vi "Weather Parse Test.vi"() -> ()   [LabVIEW 2020, in "CDM-Config.lvlib"] (continued)
                \"073355\"\n                    ],\n                    \"UGC\": [\n                        \"ANZ355\"\n                    ]\n                },\n                \"affectedZones\": [\n                    \"https://api.weather.gov/zones/forecast/ANZ355\"\n                ],\n                \"references\": [\n                    {\n                        \"@id\": \"https://api.weather.gov/alerts/urn:oid:2.49.0.1.840.0.65e698b6ba470dcf13b408ab2bfb144a0f90de6e.002.1\",\n                        \"identifier\": \"urn:oid:2.49.0.1.840.0.65e698b6ba470dcf13b408ab2bfb144a0f90de6e.002.1\",\n                        \"sender\": \"w-nws.webmaster@noaa.gov\",\n                        \"sent\": \"2025-12-03T03:02:00-05:00\"\n                    }\n                ],\n                \"sent\": \"2025-12-03T06:40:00-05:00\",\n                \"effective\": \"2025-12-03T06:40:00-05:00\",\n                \"onset\": \"2025-12-03T06:40:00-05:00\",\n                \"expires\": \"2025-12-03T12:00:00-05:00\",\n                \"ends\": \"2025-12-03T12:00:00-05:00\",\n                \"status\": \"Actual\",\n                \"messageType\": \"Update\",\n                \"category\": \"Met\",\n                \"severity\": \"Minor\",\n                \"certainty\": \"Likely\",\n                \"urgency\": \"Expected\",\n                \"event\": \"Small Craft Advisory\",\n                \"sender\": \"w-nws.webmaster@noaa.gov\",\n                \"senderName\": \"NWS Upton NY\",\n                \"headline\": \"Small Craft Advisory issued December 3 at 6:40AM EST until December 3 at 12:00PM EST by NWS Upton NY\",\n                \"description\": \"* WHAT...Northwest winds 10 to 20 kt with gusts up to 25 kt and\\nseas 3 to 5 feet.\\n\\n* WHERE...Sandy Hook NJ to Fire Island Inlet NY out 20 nm.\\n\\n* WHEN...Until noon EST today.\\n\\n* IMPACTS...Conditions will be hazardous to small craft.\",\n                \"instruction\": \"Inexperienced mariners, especially those operating smaller\\nvessels, should avoid navigating in hazardous conditions.\",\n                \"response\": \"Avoid\",\n                \"parameters\": {\n                    \"AWIPSidentifier\": [\n                        \"MWWOKX\"\n                    ],\n                    \"WMOidentifier\": [\n                        \"WHUS71 KOKX 031140\"\n                    ],\n                    \"NWSheadline\": [\n                        \"SMALL CRAFT ADVISORY REMAINS IN EFFECT UNTIL NOON EST TODAY\"\n                    ],\n                    \"BLOCKCHANNEL\": [\n                        \"EAS\",\n                        \"NWEM\",\n                        \"CMAS\"\n                    ],\n                    \"VTEC\": [\n                        \"/O.CON.KOKX.SC.Y.0111.000000T0000Z-251203T1700Z/\"\n                    ],\n                    \"eventEndingTime\": [\n                        \"2025-12-03T12:00:00-05:00\"\n                    ],\n                    \"expiredReferences\": [\n                        \"w-nws.webmaster@noaa.gov,urn:oid:2.49.0.1.840.0.ccba0ca9284c1e638a678cfbb9d4c4131fa82910.003.1,2025-12-02T13:01:00-05:00 w-nws.webmaster@noaa.gov,urn:oid:2.49.0.1.840.0.f66193c09c556463d3d8c63bce1b034f3b0ce6c5.001.1,2025-12-02T01:36:00-05:00 w-nws.webmaster@noaa.gov,urn:oid:2.49.0.1.840.0.57e44e37368416f721b2e96097448da44f0e554e.001.2,2025-12-01T13:22:00-05:00\"\n                    ]\n                },\n                \"scope\": \"Public\",\n                \"code\": \"IPAWSv1.0\",\n                \"language\": \"en-US\",\n                \"web\": \"http://www.weather.gov\",\n                \"eventCode\": {\n                    \"SAME\": [\n                        \"NWS\"\n                    ],\n                    \"NationalWeatherService\": [\n                        \"SCY\"\n                    ]\n                }\n            }\n        },\n        {\n            \"id\": \"https://api.weather.gov/alerts/urn:oid:2.49.0.1.840.0.eda6a12a51dab3b83bf60aa6decb3c42e9ebbac9.001.2\",\n            \"type\": \"Feature\",\n            \"geometry\": null,\n            \"properties\": {\n                \"@id\": \"https://api.weather.gov/alerts/urn:oid:2.49.0.1.840.0.eda6a12a51dab3b83bf60aa6decb3c42e9ebbac9.001.2\",\n                \"@type\": \"wx:Alert\",\n                \"id\": \"urn:oid:2.49.0.1.840.0.eda6a12a51dab3b83bf60aa6decb3c42e9ebbac9.001.2\",\n                \"areaDesc\": \"Moriches Inlet NY to Montauk Point NY out 20 nm; Fire Island Inlet NY to Moriches Inlet NY out 20 nm\",\n                \"geocode\": {\n                    \"SAME\": [\n                        \"073350\",\n                        \"073353\"\n                    ],\n                    \"UGC\": [\n                        \"ANZ350\",\n                        \"ANZ353\"\n                    ]\n                },\n                \"affectedZones\": [\n                    \"https://api.weather.gov/zones/forecast/ANZ350\",\n                    \"https://api.weather.gov/zones/forecast/ANZ353\"\n                ],\n                \"references\": [\n                    {\n                        \"@id\": \"https://api.weather.gov/alerts/urn:oid:2.49.0.1.840.0.65e698b6ba470dcf13b408ab2bfb144a0f90de6e.001.2\",\n                        \"identifier\": \"urn:oid:2.49.0.1.840.0.65e698b6ba470dcf13b408ab2bfb144a0f90de6e.001.2\",\n                        \"sender\": \"w-nws.webmaster@noaa.gov\",\n                        \"sent\": \"2025-12-03T03:02:00-05:00\"\n                    }\n                ],\n                \"sent\": \"2025-12-03T06:40:00-05:00\",\n                \"effective\": \"2025-12-03T06:40:00-05:00\",\n                \"onset\": \"2025-12-04T15:00:00-05:00\",\n                \"expires\": \"2025-12-03T19:45:00-05:00\",\n                \"ends\": \"2025-12-05T06:00:00-05:00\",\n                \"status\": \"Actual\",\n                \"messageType\": \"Update\",\n                \"category\": \"Met\",\n                \"severity\": \"Moderate\",\n                \"certainty\": \"Possible\",\n                \"urgency\": \"Future\",\n                \"event\": \"Gale Watch\",\n                \"sender\": \"w-nws.webmaster@noaa.gov\",\n                \"senderName\": \"NWS Upton NY\",\n                \"headline\": \"Gale Watch issued December 3 at 6:40AM EST until December 5 at 6:00AM EST by NWS Upton NY\",\n                \"description\": \"* WHAT...For the Small Craft Advisory, west winds 15 to 20 kt with\\ngusts up to 25 kt and seas 4 to 7 feet. For the Gale Watch,\\nnorthwest winds 20 to 30 kt with gusts up to 40 kt and seas 5 to\\n8 feet possible.\\n\\n* WHERE...Fire Island Inlet NY to Montauk Point NY out 20 nm.\\n\\n* WHEN...For the Small Craft Advisory, until 3 PM EST Thursday.\\nFor the Gale Watch, from Thursday afternoon through late\\nThursday night.\\n\\n* IMPACTS...Strong winds can cause hazardous seas which could\\ncapsize or damage vessels and reduce visibility.\",\n                \"instruction\": \"Mariners should consider altering plans to avoid possible\\nhazardous conditions.  Remain in port, seek safe harbor, alter\\ncourse, and/or secure the vessel for severe wind and seas.\",\n                \"response\": \"Prepare\",\n                \"parameters\": {\n                    \"AWIPSidentifier\": [\n                        \"MWWOKX\"\n                    ],\n                    \"WMOidentifier\": [\n                        \"WHUS71 KOKX 031140\"\n                    ],\n                    \"NWSheadline\": [\n                        \"SMALL CRAFT ADVISORY REMAINS IN EFFECT UNTIL 3 PM EST THURSDAY... ...GALE WATCH REMAINS IN EFFECT FROM THURSDAY AFTERNOON THROUGH LATE THURSDAY NIGHT\"\n                    ],\n                    \"BLOCKCHANNEL\": [\n                        \"EAS\",\n                        \"NWEM\",\n                        \"CMAS\"\n                    ],\n                    \"VTEC\": [\n                        \"/O.CON.KOKX.GL.A.0021.251204T2000Z-251205T1100Z/\"\n                    ],\n                    \"eventEndingTime\": [\n                        \"2025-12-05T06:00:00-05:00\"\n                    ]\n                },\n                \"scope\": \"Public\",\n                \"code\": \"IPAWSv1.0\",\n                \"language\": \"en-US\",\n                \"web\": \"http://www.weather.gov\",\n                \"eventCode\": {\n                    \"SAME\": [\n                        \"NWS\"\n                    ],\n                    \"NationalWeatherService\": [\n                        \"GLA\"\n                    ]\n                }\n            }\n        },\n        {\n            \"id\": \"https://api.weather.gov/alerts/urn:oid:2.49.0.1.840.0.0d83c610c5424770356d8de2248dc8d571fcc2f4.001.1\",\n            \"type\": \"Feature\",\n            \"geometry\": null,\n            \"properties\": {\n                \"@id\": \"https://api.weather.gov/alerts/urn:oid:2.49.0.1.840.0.0d83c610c5424770356d8de2248dc8d571fcc2f4.001.1\",\n                \"@type\": \"wx:Alert\",\n                \"id\": \"urn:oid:2.49.0.1.840.0.0d83c610c5424770356d8de2248dc8d571fcc2f4.001.1\",\n                \"areaDesc\": \"Foothills of the Northern Blue Mountains of Oregon; Yakima Valley; Foothills of the Blue Mountains of Washington\",\n                \"geocode\": {\n                    \"SAME\": [\n                        \"041059\",\n                        \"053077\",\n                        \"053013\",\n                        \"053071\"\n                    ],\n                    \"UGC\": [\n                        \"ORZ507\",\n                        \"WAZ027\",\n                        \"WAZ029\"\n                    ]\n                },\n                \"affectedZones\": [\n                    \"https://api.weather.gov/zones/forecast/ORZ507\",\n                    \"https://api.weather.gov/zones/forecast/WAZ027\",\n                    \"https://api.weather.gov/zones/forecast/WAZ029\"\n                ],\n                \"references\": [],\n                \"sent\": \"2025-12-03T02:34:00-08:00\",\n                \"effective\": \"2025-12-03T02:34:00-08:00\",\n                \"onset\": \"2025-12-03T02:34:00-08:00\",\n                \"expires\": \"2025-12-03T10:00:00-08:00\",\n                \"ends\": \"2025-12-03T10:00:00-08:00\",\n                \"status\": \"Actual\",\n                \"messageType\": \"Alert\",\n                \"category\": \"Met\",\n                \"severity\": \"Moderate\",\n                \"certainty\": \"Likely\",\n                \"urgency\": \"Expected\",\n                \"event\": \"Freezing Fog Advisory\",\n                \"sender\": \"w-nws.webmaster@noaa.gov\",\n                \"senderName\": \"NWS Pendleton OR\",\n                \"headline\": \"Freezing Fog Advisory issued December 3 at 2:34AM PST until December 3 at 10:00AM PST by NWS Pendleton OR\",\n                \"description\": \"* WHAT...Visibility generally between one-half mile and one mile in\\nfog and freezing fog.\\n\\n* WHERE...In Oregon, Foothills of the Northern Blue Mountains of\\nOregon. In Washington, Yakima Valley and Foothills of the Blue\\nMountains of Washington.\\n\\n* WHEN...Until 10 AM PST this morning.\\n\\n* IMPACTS...Low visibility could make driving conditions hazardous.\\n\\n* ADDITIONAL DETAILS...Webcams show reduced visibilities on portions\\nof I-84, SR-204 and SR-11 near Pendleton, Athena and Walla Walla\\nand SR-24 and I-82 between Sunnyside and Yakima.\",\n                \"instruction\": \"If driving, slow down, use low beam headlights, and leave plenty of\\ndistance ahead of you.\",\n                \"response\": \"Avoid\",\n                \"parameters\": {\n                    \"AWIPSidentifier\": [\n                        \"NPWPDT\"\n                    ],\n                    \"WMOidentifier\": [\n                        \"WWUS76 KPDT 031034\"\n                    ],\n                    \"NWSheadline\": [\n                        \"FREEZING FOG ADVISORY IN EFFECT UNTIL 10 AM PST THIS MORNING\"\n                    ],\n                    \"BLOCKCHANNEL\": [\n                        \"EAS\",\n                        \"NWEM\",\n                        \"CMAS\"\n                    ],\n                    \"VTEC\": [\n                        \"/O.NEW.KPDT.ZF.Y.0011.251203T1034Z-251203T1800Z/\"\n                    ],\n                    \"eventEndingTime\": [\n                        \"2025-12-03T10:00:00-08:00\"\n                    ]\n                },\n                \"scope\": \"Public\",\n                \"code\": \"IPAWSv1.0\",\n                \"language\": \"en-US\",\n                \"web\": \"http://www.weather.gov\",\n                \"eventCode\": {\n                    \"SAME\": [\n                        \"NWS\"\n                    ],\n                    \"NationalWeatherService\": [\n                        \"ZFY\"\n                    ]\n                }\n            }\n        },\n        {\n            \"id\": \"https://api.weather.gov/alerts/urn:oid:2.49.0.1.840.0.15f495c3cdd4a42513043897320797e7c1790118.004.1\",\n            \"type\": \"Feature\",\n            \"geometry\": null,\n            \"properties\": {\n                \"@id\": \"https://api.weather.gov/alerts/urn:oid:2.49.0.1.840.0.15f495c3cdd4a42513043897320797e7c1790118.004.1\",\n                \"@type\": \"wx:Alert\",\n                \"id\": \"urn:oid:2.49.0.1.840.0.15f495c3cdd4a42513043897320797e7c1790118.004.1\",\n                \"areaDesc\": \"Waters from Point Pinos to Point Piedras Blancas 10-60 NM\",\n                \"geocode\": {\n                    \"SAME\": [\n                        \"057576\"\n                    ],\n                    \"UGC\": [\n                        \"PZZ576\"\n                    ]\n                },\n                \"affectedZones\": [\n                    \"https://api.weather.gov/zones/forecast/PZZ576\"\n                ],\n                \"references\": [\n                    {\n                        \"@id\": \"https://api.weather.gov/alerts/urn:oid:2.49.0.1.840.0.2e2b4d19d93828c0d7fe64253ee2ca5ea893eca3.004.1\",\n                        \"identifier\": \"urn:oid:2.49.0.1.840.0.2e2b4d19d93828c0d7fe64253ee2ca5ea893eca3.004.1\",\n                        \"sender\": \"w-nws.webmaster@noaa.gov\",\n                        \"sent\": \"2025-12-02T20:09:00-08:00\"\n                    }\n                ],\n                \"sent\": \"2025-12-03T02:34:00-08:00\",\n                \"effective\": \"2025-12-03T02:34:00-08:00\",\n                \"onset\": \"2025-12-03T02:34:00-08:00\",\n                \"expires\": \"2025-12-03T09:00:00-08:00\",\n                \"ends\": \"2025-12-03T09:00:00-08:00\",\n                \"status\": \"Actual\",\n                \"messageType\": \"Update\",\n                \"category\": \"Met\",\n                \"severity\": \"Minor\",\n                \"certainty\": \"Likely\",\n                \"urgency\": \"Expected\",\n                \"event\": \"Small Craft Advisory\",\n                \"sender\": \"w-nws.webmaster@noaa.gov\",\n                \"senderName\": \"NWS San Francisco CA\",\n                \"headline\": \"Small Craft Advisory issued December 3 at 2:34AM PST until December 3 at 9:00AM PST by NWS San Francisco CA\",\n                \"description\": \"* WHAT...North winds 15 to 20 kt with gusts up to 30 kt and seas\\n8 to 10 ft.\\n\\n* WHERE...Waters from Point Pinos to Point Piedras Blancas 10-\\n60 NM.\\n\\n* WHEN...Until 9 AM PST this morning.\\n\\n* IMPACTS...Conditions will be hazardous to small craft.\",\n                \"instruction\": \"Inexperienced mariners, especially those operating smaller\\nvessels, should avoid navigating in hazardous conditions.\",\n                \"response\": \"Avoid\",\n                \"parameters\": {\n                    \"AWIPSidentifier\": [\n                        \"MWWMTR\"\n                    ],\n                    \"WMOidentifier\": [\n                        \"WHUS76 KMTR 031034\"\n                    ],\n                    \"NWSheadline\": [\n                        \"SMALL CRAFT ADVISORY NOW IN EFFECT UNTIL 9 AM PST THIS MORNING\"\n                    ],\n                    \"BLOCKCHANNEL\": [\n                        \"EAS\",\n                        \"NWEM\",\n                        \"CMAS\"\n                    ],\n                    \"VTEC\": [\n                        \"/O.EXT.KMTR.SC.Y.0211.000000T0000Z-251203T1700Z/\"\n                    ],\n                    \"eventEndingTime\": [\n                        \"2025-12-03T09:00:00-08:00\"\n                    ],\n                    \"expiredReferences\": [\n                        \"w-nws.webmaster@noaa.gov,urn:oid:2.49.0.1.840.0.9218f4c28c3a850a1d7ea8eb0351e78dfe99a87f.003.1,2025-12-02T14:32:00-08:00 w-nws.webmaster@noaa.gov,urn:oid:2.49.0.1.840.0.0694ec14bef3aec9c3b54940004682f896b5d224.006.1,2025-12-02T08:49:00-08:00 w-nws.webmaster@noaa.gov,urn:oid:2.49.0.1.840.0.917c99b05a9fd34906c56c3461dc077eb8fbc6c3.005.1,2025-12-02T02:30:00-08:00 w-nws.webmaster@noaa.gov,urn:oid:2.49.0.1.840.0.71e8f8c0a9680225e124435739f52670c4652e60.005.1,2025-12-01T20:36:00-08:00 w-nws.webmaster@noaa.gov,urn:oid:2.49.0.1.840.0.dc88dd948d918d864c0dc5e6ad60facca6edd43a.003.1,2025-12-01T14:02:00-08:00\"\n                    ]\n                },\n                \"scope\": \"Public\",\n                \"code\": \"IPAWSv1.0\",\n                \"language\": \"en-US\",\n                \"web\": \"http://www.weather.gov\",\n                \"eventCode\": {\n                    \"SAME\": [\n                        \"NWS\"\n                    ],\n                    \"NationalWeatherService\": [\n                        \"SCY\"\n                    ]\n                }\n            }\n        },\n        {\n            \"id\": \"https://api.weather.gov/alerts/urn:oid:2.49.0.1.840.0.15f495c3cdd4a42513043897320797e7c1790118.003.1\",\n            \"type\": \"Feature\",\n            \"geometry\": null,\n            \"properties\": {\n                \"@id\": \"https://api.weather.gov/alerts/urn:oid:2.49.0.1.840.0.15f495c3cdd4a42513043897320797e7c1790118.003.1\",\n                \"@type\": \"wx:Alert\",\n                \"id\": \"urn:oid:2.49.0.1.840.0.15f495c3cdd4a42513043897320797e7c1790118.003.1\",\n                \"areaDesc\": \"Waters from Point Reyes to Pigeon Point 10-60 NM\",\n                \"geocode\": {\n                    \"SAME\": [\n                        \"057571\"\n                    ],\n                    \"UGC\": [\n                        \"PZZ571\"\n                    ]\n                },\n                \"affectedZones\": [\n                    \"https://api.weather.gov/zones/forecast/PZZ571\"\n                ],\n                \"references\": [\n                    {\n                        \"@id\": \"https://api.weather.gov/alerts/urn:oid:2.49.0.1.840.0.2e2b4d19d93828c0d7fe64253ee2ca5ea893eca3.002.1\",\n                        \"identifier\": \"urn:oid:2.49.0.1.840.0.2e2b4d19d93828c0d7fe64253ee2ca5ea893eca3.002.1\",\n                        \"sender\": \"w-nws.webmaster@noaa.gov\",\n                        \"sent\": \"2025-12-02T20:09:00-08:00\"\n                    }\n                ],\n                \"sent\": \"2025-12-03T02:34:00-08:00\",\n                \"effective\": \"2025-12-03T02:34:00-08:00\",\n                \"onset\": \"2025-12-03T02:34:00-08:00\",\n                \"expires\": \"2025-12-03T10:45:00-08:00\",\n                \"ends\": \"2025-12-03T09:00:00-08:00\",\n                \"status\": \"Actual\",\n                \"messageType\": \"Update\",\n                \"category\": \"Met\",\n                \"severity\": \"Minor\",\n                \"certainty\": \"Likely\",\n                \"urgency\": \"Expected\",\n                \"event\": \"Small Craft Advisory\",\n                \"sender\": \"w-nws.webmaster@noaa.gov\",\n                \"senderName\": \"NWS San Francisco CA\",\n                \"headline\": \"Small Craft Advisory issued December 3 at 2:34AM PST until December 3 at 9:00AM PST by NWS San Francisco CA\",\n                \"description\": \"* WHAT...For the first Small Craft Advisory, north winds 10 to\\n20 kt with gusts up to 30 kt and seas 8 to 11 ft. For the\\nsecond Small Craft Advisory, northwest winds 10 to 20 kt with\\ngusts up to 30 kt expected.\\n\\n* WHERE...Waters from Point Reyes to Pigeon Point 10-60 NM.\\n\\n* WHEN...For the first Small Craft Advisory, until 9 AM PST this\\nmorning. For the second Small Craft Advisory, from 9 PM\\nThursday to 9 AM PST Friday.\\n\\n* IMPACTS...Conditions will be hazardous to small craft.\",\n                \"instruction\": \"Inexperienced mariners, especially those operating smaller\\nvessels, should avoid navigating in hazardous conditions.\",\n                \"response\": \"Avoid\",\n                \"parameters\": {\n                    \"AWIPSidentifier\": [\n                        \"MWWMTR\"\n                    ],\n                    \"WMOidentifier\": [\n                        \"WHUS76 KMTR 031034\"\n                    ],\n                    \"NWSheadline\": [\n                        \"SMALL CRAFT ADVISORY REMAINS IN EFFECT UNTIL 9 AM PST THIS MORNING... ...SMALL CRAFT ADVISORY IN EFFECT FROM 9 PM THURSDAY TO 9 AM PST FRIDAY\"\n                    ],\n                    \"BLOCKCHANNEL\": [\n                        \"EAS\",\n                        \"NWEM\",\n                        \"CMAS\"\n                    ],\n                    \"VTEC\": [\n                        \"/O.CON.KMTR.SC.Y.0210.000000T0000Z-251203T1700Z/\"\n                    ],\n                    \"eventEndingTime\": [\n                        \"2025-12-03T09:00:00-08:00\"\n                    ],\n                    \"expiredReferences\": [\n                        \"w-nws.webmaster@noaa.gov,urn:oid:2.49.0.1.840.0.9218f4c28c3a850a1d7ea8eb0351e78dfe99a87f.004.1,2025-12-02T14:32:00-08:00 w-nws.webmaster@noaa.gov,urn:oid:2.49.0.1.840.0.0694ec14bef3aec9c3b54940004682f896b5d224.003.1,2025-12-02T08:49:00-08:00 w-nws.webmaster@noaa.gov,urn:oid:2.49.0.1.840.0.917c99b05a9fd34906c56c3461dc077eb8fbc6c3.003.1,2025-12-02T02:30:00-08:00 w-nws.webmaster@noaa.gov,urn:oid:2.49.0.1.840.0.71e8f8c0a9680225e124435739f52670c4652e60.002.1,2025-12-01T20:36:00-08:00 w-nws.webmaster@noaa.gov,urn:oid:2.49.0.1.840.0.dc88dd948d918d864c0dc5e6ad60facca6edd43a.004.1,2025-12-01T14:02:00-08:00\"\n                    ]\n                },\n                \"scope\": \"Public\",\n                \"code\": \"IPAWSv1.0\",\n                \"language\": \"en-US\",\n                \"web\": \"http://www.weather.gov\",\n                \"eventCode\": {\n                    \"SAME\": [\n                        \"NWS\"\n                    ],\n                    \"NationalWeatherService\": [\n                        \"SCY\"\n                    ]\n                }\n            }\n        },\n        {\n            \"id\": \"https://api.weather.gov/alerts/urn:oid:2.49.0.1.840.0.15f495c3cdd4a42513043897320797e7c1790118.003.2\",\n            \"type\": \"Feature\",\n            \"geometry\": null,\n            \"properties\": {\n                \"@id\": \"https://api.weather.gov/alerts/urn:oid:2.49.0.1.840.0.15f495c3cdd4a42513043897320797e7c1790118.003.2\",\n                \"@type\": \"wx:Alert\",\n                \"id\": \"urn:oid:2.49.0.1.840.0.15f495c3cdd4a42513043897320797e7c1790118.003.2\",\n                \"areaDesc\": \"Waters from Point Reyes to Pigeon Point 10-60 NM\",\n                \"geocode\": {\n                    \"SAME\": [\n                        \"057571\"\n                    ],\n                    \"UGC\": [\n                        \"PZZ571\"\n                    ]\n                },\n                \"affectedZones\": [\n                    \"https://api.weather.gov/zones/forecast/PZZ571\"\n                ],\n                \"references\": [],\n                \"sent\": \"2025-12-03T02:34:00-08:00\",\n                \"effective\": \"2025-12-03T02:34:00-08:00\",\n                \"onset\": \"2025-12-04T21:00:00-08:00\",\n                \"expires\": \"2025-12-03T10:45:00-08:00\",\n                \"ends\": \"2025-12-05T09:00:00-08:00\",\n                \"status\": \"Actual\",\n                \"messageType\": \"Alert\",\n                \"category\": \"Met\",\n                \"severity\": \"Minor\",\n                \"certainty\": \"Likely\",\n                \"urgency\": \"Expected\",\n                \"event\": \"Small Craft Advisory\",\n                \"sender\": \"w-nws.webmaster@noaa.gov\",\n                \"senderName\": \"NWS San Francisco CA\",\n                \"headline\": \"Small Craft Advisory issued December 3 at 2:34AM PST until December 5 at 9:00AM PST by NWS San Francisco CA\",\n                \"description\": \"* WHAT...For the first Small Craft Advisory, north winds 10 to\\n20 kt with gusts up to 30 kt and seas 8 to 11 ft. For the\\nsecond Small Craft Advisory, northwest winds 10 to 20 kt with\\ngusts up to 30 kt expected.\\n\\n* WHERE...Waters from Point Reyes to Pigeon Point 10-60 NM.\\n\\n* WHEN...For the first Small Craft Advisory, until 9 AM PST this\\nmorning. For the second Small Craft Advisory, from 9 PM\\nThursday to 9 AM PST Friday.\\n\\n* IMPACTS...Conditions will be hazardous to small craft.\",\n                \"instruction\": \"Inexperienced mariners, especially those operating smaller\\nvessels, should avoid navigating in hazardous conditions.\",\n                \"response\": \"Avoid\",\n                \"parameters\": {\n                    \"AWIPSidentifier\": [\n                        \"MWWMTR\"\n                    ],\n                    \"WMOidentifier\": [\n                        \"WHUS76 KMTR 031034\"\n                    ],\n                    \"NWSheadline\": [\n                        \"SMALL CRAFT ADVISORY REMAINS IN EFFECT UNTIL 9 AM PST THIS MORNING... ...SMALL CRAFT ADVISORY IN EFFECT FROM 9 PM THURSDAY TO 9 AM PST FRIDAY\"\n                    ],\n                    \"BLOCKCHANNEL\": [\n                        \"EAS\",\n                        \"NWEM\",\n                        \"CMAS\"\n                    ],\n                    \"VTEC\": [\n                        \"/O.NEW.KMTR.SC.Y.0212.251205T0500Z-251205T1700Z/\"\n                    ],\n                    \"eventEndingTime\": [\n                        \"2025-12-05T09:00:00-08:00\"\n                    ]\n                },\n                \"scope\": \"Public\",\n                \"code\": \"IPAWSv1.0\",\n                \"language\": \"en-US\",\n                \"web\": \"http://www.weather.gov\",\n                \"eventCode\": {\n                    \"SAME\": [\n                        \"NWS\"\n                    ],\n                    \"NationalWeatherService\": [\n                        \"SCY\"\n                    ]\n                }\n            }\n        },\n        {\n            \"id\": \"https://api.weather.gov/alerts/urn:oid:2.49.0.1.840.0.15f495c3cdd4a42513043897320797e7c1790118.002.2\",\n            \"type\": \"Feature\",\n            \"geometry\": null,\n            \"properties\": {\n                \"@id\": \"https://api.weather.gov/alerts/urn:oid:2.49.0.1.840.0.15f495c3cdd4a42513043897320797e7c1790118.002.2\",\n                \"@type\": \"wx:Alert\",\n                \"id\": \"urn:oid:2.49.0.1.840.0.15f495c3cdd4a42513043897320797e7c1790118.002.2\",\n                \"areaDesc\": \"Waters from Point Arena to Point Reyes 10-60 NM\",\n                \"geocode\": {\n                    \"SAME\": [\n                        \"057570\"\n                    ],\n                    \"UGC\": [\n                        \"PZZ570\"\n                    ]\n                },\n                \"affectedZones\": [\n                    \"https://api.weather.gov/zones/forecast/PZZ570\"\n                ],\n                \"references\": [],\n                \"sent\": \"2025-12-03T02:34:00-08:00\",\n                \"effective\": \"2025-12-03T02:34:00-08:00\",\n                \"onset\": \"2025-12-04T21:00:00-08:00\",\n                \"expires\": \"2025-12-03T10:45:00-08:00\",\n                \"ends\": \"2025-12-05T09:00:00-08:00\",\n                \"status\": \"Actual\",\n                \"messageType\": \"Alert\",\n                \"category\": \"Met\",\n                \"severity\": \"Minor\",\n                \"certainty\": \"Likely\",\n                \"urgency\": \"Expected\",\n                \"event\": \"Small Craft Advisory\",\n                \"sender\": \"w-nws.webmaster@noaa.gov\",\n                \"senderName\": \"NWS San Francisco CA\",\n                \"headline\": \"Small Craft Advisory issued December 3 at 2:34AM PST until December 5 at 9:00AM PST by NWS San Francisco CA\",\n                \"description\": \"* WHAT...For the first Small Craft Advisory, north winds 15 to\\n25 kt with gusts up to 35 kt and seas 8 to 11 ft. For the\\nsecond Small Craft Advisory, north winds 15 to 25 kt with\\ngusts up to 30 kt expected.\\n\\n* WHERE...Waters from Point Arena to Point Reyes 10-60 NM.\\n\\n* WHEN...For the first Small Craft Advisory, until 3 PM PST this\\nafternoon. For the second Small Craft Advisory, from 9 PM\\nThursday to 9 AM PST Friday.\\n\\n* IMPACTS...Conditions will be hazardous to small craft.\",\n                \"instruction\": \"Inexperienced mariners, especially those operating smaller\\nvessels, should avoid navigating in hazardous conditions.\",\n                \"response\": \"Avoid\",\n                \"parameters\": {\n                    \"AWIPSidentifier\": [\n                        \"MWWMTR\"\n                    ],\n                    \"WMOidentifier\": [\n                        \"WHUS76 KMTR 031034\"\n                    ],\n                    \"NWSheadline\": [\n                        \"SMALL CRAFT ADVISORY REMAINS IN EFFECT UNTIL 3 PM PST THIS AFTERNOON... ...SMALL CRAFT ADVISORY IN EFFECT FROM 9 PM THURSDAY TO 9 AM PST FRIDAY\"\n                    ],\n                    \"BLOCKCHANNEL\": [\n                        \"EAS\",\n                        \"NWEM\",\n                        \"CMAS\"\n                    ],\n                    \"VTEC\": [\n                        \"/O.NEW.KMTR.SC.Y.0212.251205T0500Z-251205T1700Z/\"\n                    ],\n                    \"eventEndingTime\": [\n                        \"2025-12-05T09:00:00-08:00\"\n                    ]\n                },\n                \"scope\": \"Public\",\n                \"code\": \"IPAWSv1.0\",\n                \"language\": \"en-US\",\n                \"web\": \"http://www.weather.gov\",\n                \"eventCode\": {\n                    \"SAME\": [\n                        \"NWS\"\n                    ],\n                    \"NationalWeatherService\": [\n                        \"SCY\"\n                    ]\n                }\n            }\n        },\n        {\n            \"id\": \"https://api.weather.gov/alerts/urn:oid:2.49.0.1.840.0.15f495c3cdd4a42513043897320797e7c1790118.002.1\",\n            \"type\": \"Feature\",\n            \"geometry\": null,\n            \"properties\": {\n                \"@id\": \"https://api.weather.gov/alerts/urn:oid:2.49.0.1.840.0.15f495c3cdd4a42513043897320797e7c1790118.002.1\",\n                \"@type\": \"wx:Alert\",\n                \"id\": \"urn:oid:2.49.0.1.840.0.15f495c3cdd4a42513043897320797e7c1790118.002.1\",\n                \"areaDesc\": \"Waters from Point Arena to Point Reyes 10-60 NM\",\n                \"geocode\": {\n                    \"SAME\": [\n                        \"057570\"\n                    ],\n                    \"UGC\": [\n                        \"PZZ570\"\n                    ]\n                },\n                \"affectedZones\": [\n                    \"https://api.weather.gov/zones/forecast/PZZ570\"\n                ],\n                \"references\": [\n                    {\n                        \"@id\": \"https://api.weather.gov/alerts/urn:oid:2.49.0.1.840.0.2e2b4d19d93828c0d7fe64253ee2ca5ea893eca3.001.1\",\n                        \"identifier\": \"urn:oid:2.49.0.1.840.0.2e2b4d19d93828c0d7fe64253ee2ca5ea893eca3.001.1\",\n                        \"sender\": \"w-nws.webmaster@noaa.gov\",\n                        \"sent\": \"2025-12-02T20:09:00-08:00\"\n                    }\n                ],\n                \"sent\": \"2025-12-03T02:34:00-08:00\",\n                \"effective\": \"2025-12-03T02:34:00-08:00\",\n                \"onset\": \"2025-12-03T02:34:00-08:00\",\n                \"expires\": \"2025-12-03T10:45:00-08:00\",\n                \"ends\": \"2025-12-03T15:00:00-08:00\",\n                \"status\": \"Actual\",\n                \"messageType\": \"Update\",\n                \"category\": \"Met\",\n                \"severity\": \"Minor\",\n                \"certainty\": \"Likely\",\n                \"urgency\": \"Expected\",\n                \"event\": \"Small Craft Advisory\",\n                \"sender\": \"w-nws.webmaster@noaa.gov\",\n                \"senderName\": \"NWS San Francisco CA\",\n                \"headline\": \"Small Craft Advisory issued December 3 at 2:34AM PST until December 3 at 3:00PM PST by NWS San Francisco CA\",\n                \"description\": \"* WHAT...For the first Small Craft Advisory, north winds 15 to\\n25 kt with gusts up to 35 kt and seas 8 to 11 ft. For the\\nsecond Small Craft Advisory, north winds 15 to 25 kt with\\ngusts up to 30 kt expected.\\n\\n* WHERE...Waters from Point Arena to Point Reyes 10-60 NM.\\n\\n* WHEN...For the first Small Craft Advisory, until 3 PM PST this\\nafternoon. For the second Small Craft Advisory, from 9 PM\\nThursday to 9 AM PST Friday.\\n\\n* IMPACTS...Conditions will be hazardous to small craft.\",\n                \"instruction\": \"Inexperienced mariners, especially those operating smaller\\nvessels, should avoid navigating in hazardous conditions.\",\n                \"response\": \"Avoid\",\n                \"parameters\": {\n                    \"AWIPSidentifier\": [\n                        \"MWWMTR\"\n                    ],\n                    \"WMOidentifier\": [\n                        \"WHUS76 KMTR 031034\"\n                    ],\n                    \"NWSheadline\": [\n                        \"SMALL CRAFT ADVISORY REMAINS IN EFFECT UNTIL 3 PM PST THIS AFTERNOON... ...SMALL CRAFT ADVISORY IN EFFECT FROM 9 PM THURSDAY TO 9 AM PST FRIDAY\"\n                    ],\n                    \"BLOCKCHANNEL\": [\n                        \"EAS\",\n                        \"NWEM\",\n                        \"CMAS\"\n                    ],\n                    \"VTEC\": [\n                        \"/O.CON.KMTR.SC.Y.0211.000000T0000Z-251203T2300Z/\"\n                    ],\n                    \"eventEndingTime\": [\n                        \"2025-12-03T15:00:00-08:00\"\n                    ],\n                    \"expiredReferences\": [\n                        \"w-nws.webmaster@noaa.gov,urn:oid:2.49.0.1.840.0.9218f4c28c3a850a1d7ea8eb0351e78dfe99a87f.001.3,2025-12-02T14:32:00-08:00\"\n                    ]\n                },\n                \"scope\": \"Public\",\n                \"code\": \"IPAWSv1.0\",\n                \"language\": \"en-US\",\n                \"web\": \"http://www.weather.gov\",\n                \"eventCode\": {\n                    \"SAME\": [\n                        \"NWS\"\n                    ],\n                    \"NationalWeatherService\": [\n                        \"SCY\"\n                    ]\n                }\n            }\n        },\n        {\n            \"id\": \"https://api.weather.gov/alerts/urn:oid:2.49.0.1.840.0.15f495c3cdd4a42513043897320797e7c1790118.005.1\",\n            \"type\": \"Feature\",\n            \"geometry\": null,\n            \"properties\": {\n                \"@id\": \"https://api.weather.gov/alerts/urn:oid:2.49.0.1.840.0.15f495c3cdd4a42513043897320797e7c1790118.005.1\",\n                \"@type\": \"wx:Alert\",\n                \"id\": \"urn:oid:2.49.0.1.840.0.15f495c3cdd4a42513043897320797e7c1790118.005.1\",\n                \"areaDesc\": \"Waters from Pigeon Point to Point Pinos 10-60 NM\",\n                \"geocode\": {\n                    \"SAME\": [\n                        \"057575\"\n                    ],\n                    \"UGC\": [\n                        \"PZZ575\"\n                    ]\n                },\n                \"affectedZones\": [\n                    \"https://api.weather.gov/zones/forecast/PZZ575\"\n                ],\n                \"references\": [\n                    {\n                        \"@id\": \"https://api.weather.gov/alerts/urn:oid:2.49.0.1.840.0.2e2b4d19d93828c0d7fe64253ee2ca5ea893eca3.003.1\",\n                        \"identifier\": \"urn:oid:2.49.0.1.840.0.2e2b4d19d93828c0d7fe64253ee2ca5ea893eca3.003.1\",\n                        \"sender\": \"w-nws.webmaster@noaa.gov\",\n                        \"sent\": \"2025-12-02T20:09:00-08:00\"\n                    }\n                ],\n                \"sent\": \"2025-12-03T02:34:00-08:00\",\n                \"effective\": \"2025-12-03T02:34:00-08:00\",\n                \"onset\": \"2025-12-03T02:34:00-08:00\",\n                \"expires\": \"2025-12-03T09:00:00-08:00\",\n                \"ends\": \"2025-12-03T09:00:00-08:00\",\n                \"status\": \"Actual\",\n                \"messageType\": \"Update\",\n                \"category\": \"Met\",\n                \"severity\": \"Minor\",\n                \"certainty\": \"Likely\",\n                \"urgency\": \"Expected\",\n                \"event\": \"Small Craft Advisory\",\n                \"sender\": \"w-nws.webmaster@noaa.gov\",\n                \"senderName\": \"NWS San Francisco CA\",\n                \"headline\": \"Small Craft Advisory issued December 3 at 2:34AM PST until December 3 at 9:00AM PST by NWS San Francisco CA\",\n                \"description\": \"* WHAT...North winds 15 to 20 kt with gusts up to 30 kt and seas\\n9 to 11 ft.\\n\\n* WHERE...Waters from Pigeon Point to Point Pinos 10-60 NM.\\n\\n* WHEN...Until 9 AM PST this morning.\\n\\n* IMPACTS...Conditions will be hazardous to small craft.\",\n                \"instruction\": \"Inexperienced mariners, especially those operating smaller\\nvessels, should avoid navigating in hazardous conditions.\",\n                \"response\": \"Avoid\",\n                \"parameters\": {\n                    \"AWIPSidentifier\": [\n                        \"MWWMTR\"\n                    ],\n                    \"WMOidentifier\": [\n                        \"WHUS76 KMTR 031034\"\n                    ],\n                    \"NWSheadline\": [\n                        \"SMALL CRAFT ADVISORY REMAINS IN EFFECT UNTIL 9 AM PST THIS MORNING\"\n                    ],\n                    \"BLOCKCHANNEL\": [\n                        \"EAS\",\n                        \"NWEM\",\n                        \"CMAS\"\n                    ],\n                    \"VTEC\": [\n                        \"/O.CON.KMTR.SC.Y.0211.000000T0000Z-251203T1700Z/\"\n                    ],\n                    \"eventEndingTime\": [\n                        \"2025-12-03T09:00:00-08:00\"\n                    ],\n                    \"expiredReferences\": [\n                        \"w-nws.webmaster@noaa.gov,urn:oid:2.49.0.1.840.0.9218f4c28c3a850a1d7ea8eb0351e78dfe99a87f.005.1,2025-12-02T14:32:00-08:00 w-nws.webmaster@noaa.gov,urn:oid:2.49.0.1.840.0.0694ec14bef3aec9c3b54940004682f896b5d224.004.1,2025-12-02T08:49:00-08:00 w-nws.webmaster@noaa.gov,urn:oid:2.49.0.1.840.0.917c99b05a9fd34906c56c3461dc077eb8fbc6c3.004.1,2025-12-02T02:30:00-08:00 w-nws.webmaster@noaa.gov,urn:oid:2.49.0.1.840.0.71e8f8c0a9680225e124435739f52670c4652e60.003.1,2025-12-01T20:36:00-08:00 w-nws.webmaster@noaa.gov,urn:oid:2.49.0.1.840.0.dc88dd948d918d864c0dc5e6ad60facca6edd43a.002.1,2025-12-01T14:02:00-08:00\"\n                    ]\n                },\n                \"scope\": \"Public\",\n                \"code\": \"IPAWSv1.0\",\n                \"language\": \"en-US\",\n                \"web\": \"http://www.weather.gov\",\n                \"eventCode\": {\n                    \"SAME\": [\n                        \"NWS\"\n                    ],\n                    \"NationalWeatherService\": [\n                        \"SCY\"\n                    ]\n                }\n            }\n        },\n        {\n            \"id\": \"https://api.weather.gov/alerts/urn:oid:2.49.0.1.840.0.f5f10ce1fc125a889b0eaa6bd36ba499c2aad555.001.1\",\n            \"type\": \"Feature\",\n            \"geometry\": null,\n            \"properties\": {\n                \"@id\": \"https://api.weather.gov/alerts/urn:oid:2.49.0.1.840.0.f5f10ce1fc125a889b0eaa6bd36ba499c2aad555.001.1\",\n                \"@type\": \"wx:Alert\",\n                \"id\": \"urn:oid:2.49.0.1.840.0.f5f10ce1fc125a889b0eaa6bd36ba499c2aad555.001.1\",\n                \"areaDesc\": \"San Diego County Coastal Areas; Orange County Coastal\",\n                \"geocode\": {\n                    \"SAME\": [\n                        \"006073\",\n                        \"006059\"\n                    ],\n                    \"UGC\": [\n                        \"CAZ043\",\n                        \"CAZ552\"\n                    ]\n                },\n                \"affectedZones\": [\n                    \"https://api.weather.gov/zones/forecast/CAZ043\",\n                    \"https://api.weather.gov/zones/forecast/CAZ552\"\n                ],\n                \"references\": [\n                    {\n                        \"@id\": \"https://api.weather.gov/alerts/urn:oid:2.49.0.1.840.0.d4f2b19dfc2ae07e10b56ffd3f205dd8244878a4.001.1\",\n                        \"identifier\": \"urn:oid:2.49.0.1.840.0.d4f2b19dfc2ae07e10b56ffd3f205dd8244878a4.001.1\",\n                        \"sender\": \"w-nws.webmaster@noaa.gov\",\n                        \"sent\": \"2025-12-02T21:21:00-08:00\"\n                    }\n                ],\n                \"sent\": \"2025-12-03T02:17:00-08:00\",\n                \"effective\": \"2025-12-03T02:17:00-08:00\",\n                \"onset\": \"2025-12-03T02:17:00-08:00\",\n                \"expires\": \"2025-12-03T14:30:00-08:00\",\n                \"ends\": \"2025-12-05T10:00:00-08:00\",\n                \"status\": \"Actual\",\n                \"messageType\": \"Update\",\n                \"category\": \"Met\",\n                \"severity\": \"Moderate\",\n                \"certainty\": \"Likely\",\n                \"urgency\": \"Expected\",\n                \"event\": \"Beach Hazards Statement\",\n                \"sender\": \"w-nws.webmaster@noaa.gov\",\n                \"senderName\": \"NWS San Diego CA\",\n                \"headline\": \"Beach Hazards Statement issued December 3 at 2:17AM PST until December 5 at 10:00AM PST by NWS San Diego CA\",\n                \"description\": \"* WHAT...Very high astronomical tides during the mornings\\ncombined with elevated surf up to 5 to 6 feet, primarily at\\nwest-facing beaches today, will result in minor tidal overflow\\nand local beach flooding.\\n\\n* WHERE...San Diego County Coastal Areas and Orange County\\nCoastal Areas.\\n\\n* WHEN...Through Friday morning.\\n\\n* IMPACTS...Minor tidal overflow, beach flooding, and coastal\\nerosion most likely during times of high tides. Hazardous\\nswimming conditions.\\n\\n* ADDITIONAL DETAILS...Predicted high tides at La Jolla: 6.8 feet\\nat 653 AM today, 7.1 feet at 734 AM Thursday, and 7.1 feet at\\n818 AM Friday.\",\n                \"instruction\": \"A beach hazards statement for minor tidal overflow means that\\nhigh astronomical tides, especially in combination with above\\nnormal surf, will likely produce minor flooding of low-lying\\nareas along the beach such as beach parking lots. Coastal\\nofficials should take the necessary precautionary measures to\\nsafeguard their beaches.\\n\\nInexperienced swimmers should remain out of the water to avoid\\nhazardous swimming conditions.\",\n                \"response\": \"Avoid\",\n                \"parameters\": {\n                    \"AWIPSidentifier\": [\n                        \"CFWSGX\"\n                    ],\n                    \"WMOidentifier\": [\n                        \"WHUS46 KSGX 031017\"\n                    ],\n                    \"NWSheadline\": [\n                        \"BEACH HAZARDS STATEMENT REMAINS IN EFFECT THROUGH FRIDAY MORNING\"\n                    ],\n                    \"BLOCKCHANNEL\": [\n                        \"EAS\",\n                        \"NWEM\",\n                        \"CMAS\"\n                    ],\n                    \"VTEC\": [\n                        \"/O.CON.KSGX.BH.S.0015.000000T0000Z-251205T1800Z/\"\n                    ],\n                    \"eventEndingTime\": [\n                        \"2025-12-05T10:00:00-08:00\"\n                    ],\n                    \"expiredReferences\": [\n                        \"w-nws.webmaster@noaa.gov,urn:oid:2.49.0.1.840.0.00a37a2404c202bcf0ae762169bc567d158b9285.001.1,2025-12-02T13:21:00-08:00 w-nws.webmaster@noaa.gov,urn:oid:2.49.0.1.840.0.be3b807b2b6a6a1bfaaf6102241c127066b8ba58.001.1,2025-12-02T02:03:00-08:00 w-nws.webmaster@noaa.gov,urn:oid:2.49.0.1.840.0.ee9a6e4ab7aa05c99a30ab57af41248485e66d1e.001.1,2025-12-01T12:12:00-08:00 w-nws.webmaster@noaa.gov,urn:oid:2.49.0.1.840.0.bd26b50bc51840d8c07e77dc2b90751ceaaad7e8.001.1,2025-12-01T12:05:00-08:00\"\n                    ]\n                },\n                \"scope\": \"Public\",\n                \"code\": \"IPAWSv1.0\",\n                \"language\": \"en-US\",\n                \"web\": \"http://www.weather.gov\",\n                \"eventCode\": {\n                    \"SAME\": [\n                        \"NWS\"\n                    ],\n                    \"NationalWeatherService\": [\n                        \"BHS\"\n                    ]\n                }\n            }\n        },\n        {\n            \"id\": \"https://api.weather.gov/alerts/urn:oid:2.49.0.1.840.0.751dc1a2e1a8739776f90401a27d104adde35eee.001.1\",\n            \"type\": \"Feature\",\n            \"geometry\": null,\n            \"properties\": {\n                \"@id\": \"https://api.weather.gov/alerts/urn:oid:2.49.0.1.840.0.751dc1a2e1a8739776f90401a27d104adde35eee.001.1\",\n                \"@type\": \"wx:Alert\",\n                \"id\": \"urn:oid:2.49.0.1.840.0.751dc1a2e1a8739776f90401a27d104adde35eee.001.1\",\n                \"areaDesc\": \"Wayne; Fayette; Union; Franklin; Ripley; Dearborn; Ohio; Switzerland; Carroll; Gallatin; Boone; Kenton; Campbell; Owen; Grant; Pendleton; Bracken; Robertson; Mason; Lewis; Hardin; Mercer; Auglaize; Darke; Shelby; Logan; Union; Delaware; Miami; Champaign; Clark; Madison; Franklin; Licking; Preble; Montgomery; Greene; Fayette; Pickaway; Fairfield; Butler; Warren; Clinton; Ross; Hocking; Hamilton; Clermont; Brown; Highland; Adams; Pike; Scioto\",\n                \"geocode\": {\n                    \"SAME\": [\n                        \"018177\",\n                        \"018041\",\n                        \"018161\",\n                        \"018047\",\n                        \"018137\",\n                        \"018029\",\n                        \"018115\",\n                        \"018155\",\n                        \"021041\",\n                        \"021077\",\n                        \"021015\",\n                        \"021117\",\n                        \"021037\",\n                        \"021187\",\n                        \"021081\",\n                        \"021191\",\n                        \"021023\",\n                        \"021201\",\n                        \"021161\",\n                        \"021135\",\n                        \"039065\",\n                        \"039107\",\n                        \"039011\",\n                        \"039037\",\n                        \"039149\",\n                        \"039091\",\n                        \"039159\",\n                        \"039041\",\n                        \"039109\",\n                        \"039021\",\n                        \"039023\",\n                        \"039097\",\n                        \"039049\",\n                        \"039089\",\n                        \"039135\",\n                        \"039113\",\n                        \"039057\",\n                        \"039047\",\n                        \"039129\",\n                        \"039045\",\n                        \"039017\",\n                        \"039165\",\n                        \"039027\",\n                        \"039141\",\n                        \"039073\",\n                        \"039061\",\n                        \"039025\",\n                        \"039015\",\n                        \"039071\",\n                        \"039001\",\n                        \"039131\",\n                        \"039145\"\n                    ],\n                    \"UGC\": [\n                        \"INZ050\",\n                        \"INZ058\",\n                        \"INZ059\",\n                        \"INZ066\",\n                        \"INZ073\",\n                        \"INZ074\",\n                        \"INZ075\",\n                        \"INZ080\",\n                        \"KYZ089\",\n                        \"KYZ090\",\n                        \"KYZ091\",\n                        \"KYZ092\",\n                        \"KYZ093\",\n                        \"KYZ094\",\n                        \"KYZ095\",\n                        \"KYZ096\",\n                        \"KYZ097\",\n                        \"KYZ098\",\n                        \"KYZ099\",\n                        \"KYZ100\",\n                        \"OHZ026\",\n                        \"OHZ034\",\n                        \"OHZ035\",\n                        \"OHZ042\",\n                        \"OHZ043\",\n                        \"OHZ044\",\n                        \"OHZ045\",\n                        \"OHZ046\",\n                        \"OHZ051\",\n                        \"OHZ052\",\n                        \"OHZ053\",\n                        \"OHZ054\",\n                        \"OHZ055\",\n                        \"OHZ056\",\n                        \"OHZ060\",\n                        \"OHZ061\",\n                        \"OHZ062\",\n                        \"OHZ063\",\n                        \"OHZ064\",\n                        \"OHZ065\",\n                        \"OHZ070\",\n                        \"OHZ071\",\n                        \"OHZ072\",\n                        \"OHZ073\",\n                        \"OHZ074\",\n                        \"OHZ077\",\n                        \"OHZ078\",\n                        \"OHZ079\",\n                        \"OHZ080\",\n                        \"OHZ081\",\n                        \"OHZ082\",\n                        \"OHZ088\"\n                    ]\n                },\n                \"affectedZones\": [\n                    \"https://api.weather.gov/zones/forecast/INZ050\",\n                    \"https://api.weather.gov/zones/forecast/INZ058\",\n                    \"https://api.weather.gov/zones/forecast/INZ059\",\n                    \"https://api.weather.gov/zones/forecast/INZ066\",\n                    \"https://api.weather.gov/zones/forecast/INZ073\",\n                    \"https://api.weather.gov/zones/forecast/INZ074\",\n                    \"https://api.weather.gov/zones/forecast/INZ075\",\n                    \"https://api.weather.gov/zones/forecast/INZ080\",\n                    \"https://api.weather.gov/zones/forecast/KYZ089\",\n                    \"https://api.weather.gov/zones/forecast/KYZ090\",\n                    \"https://api.weather.gov/zones/forecast/KYZ091\",\n                    \"https://api.weather.gov/zones/forecast/KYZ092\",\n                    \"https://api.weather.gov/zones/forecast/KYZ093\",\n                    \"https://api.weather.gov/zones/forecast/KYZ094\",\n                    \"https://api.weather.gov/zones/forecast/KYZ095\",\n                    \"https://api.weather.gov/zones/forecast/KYZ096\",\n                    \"https://api.weather.gov/zones/forecast/KYZ097\",\n                    \"https://api.weather.gov/zones/forecast/KYZ098\",\n                    \"https://api.weather.gov/zones/forecast/KYZ099\",\n                    \"https://api.weather.gov/zones/forecast/KYZ100\",\n                    \"https://api.weather.gov/zones/forecast/OHZ026\",\n                    \"https://api.weather.gov/zones/forecast/OHZ034\",\n                    \"https://api.weather.gov/zones/forecast/OHZ035\",\n                    \"https://api.weather.gov/zones/forecast/OHZ042\",\n                    \"https://api.weather.gov/zones/forecast/OHZ043\",\n                    \"https://api.weather.gov/zones/forecast/OHZ044\",\n                    \"https://api.weather.gov/zones/forecast/OHZ045\",\n                    \"https://api.weather.gov/zones/forecast/OHZ046\",\n                    \"https://api.weather.gov/zones/forecast/OHZ051\",\n                    \"https://api.weather.gov/zones/forecast/OHZ052\",\n                    \"https://api.weather.gov/zones/forecast/OHZ053\",\n                    \"https://api.weather.gov/zones/forecast/OHZ054\",\n                    \"https://api.weather.gov/zones/forecast/OHZ055\",\n                    \"https://api.weather.gov/zones/forecast/OHZ056\",\n                    \"https://api.weather.gov/zones/forecast/OHZ060\",\n                    \"https://api.weather.gov/zones/forecast/OHZ061\",\n                    \"https://api.weather.gov/zones/forecast/OHZ062\",\n                    \"https://api.weather.gov/zones/forecast/OHZ063\",\n                    \"https://api.weather.gov/zones/forecast/OHZ064\",\n                    \"https://api.weather.gov/zones/forecast/OHZ065\",\n                    \"https://api.weather.gov/zones/forecast/OHZ070\",\n                    \"https://api.weather.gov/zones/forecast/OHZ071\",\n                    \"https://api.weather.gov/zones/forecast/OHZ072\",\n                    \"https://api.weather.gov/zones/forecast/OHZ073\",\n                    \"https://api.weather.gov/zones/forecast/OHZ074\",\n                    \"https://api.weather.gov/zones/forecast/OHZ077\",\n                    \"https://api.weather.gov/zones/forecast/OHZ078\",\n                    \"https://api.weather.gov/zones/forecast/OHZ079\",\n                    \"https://api.weather.gov/zones/forecast/OHZ080\",\n                    \"https://api.weather.gov/zones/forecast/OHZ081\",\n                    \"https://api.weather.gov/zones/forecast/OHZ082\",\n                    \"https://api.weather.gov/zones/forecast/OHZ088\"\n                ],\n                \"references\": [],\n                \"sent\": \"2025-12-03T05:13:00-05:00\",\n                \"effective\": \"2025-12-03T05:13:00-05:00\",\n                \"onset\": \"2025-12-03T05:13:00-05:00\",\n                \"expires\": \"2025-12-03T13:00:00-05:00\",\n                \"ends\": null,\n                \"status\": \"Actual\",\n                \"messageType\": \"Alert\",\n                \"category\": \"Met\",\n                \"severity\": \"Moderate\",\n                \"certainty\": \"Observed\",\n                \"urgency\": \"Expected\",\n                \"event\": \"Special Weather Statement\",\n                \"sender\": \"w-nws.webmaster@noaa.gov\",\n                \"senderName\": \"NWS Wilmington OH\",\n                \"headline\": \"Special Weather Statement issued December 3 at 5:13AM EST by NWS Wilmington OH\",\n                \"description\": \"Light snow is expected to develop across the area after midnight,\\nshifting to the southeast through the predawn hours. This band of\\nlight snow will affect the Tri-State region by the Thursday\\nmorning commute, eventually pushing south of the area by mid-\\nmorning.\\n\\nMinor snow accumulations of less than an inch are expected, but\\ncold ground conditions will allow for quick accumulation on any\\nuntreated surfaces. The main impacts are expected to be reduced\\nvisibilities and some slick spots on untreated surfaces.\\n\\nMotorists should exercise caution. Plan extra time for the\\nThursday morning commute.\",\n                \"instruction\": null,\n                \"response\": \"Execute\",\n                \"parameters\": {\n                    \"AWIPSidentifier\": [\n                        \"SPSILN\"\n                    ],\n                    \"WMOidentifier\": [\n                        \"WWUS81 KILN 031013\"\n                    ],\n                    \"NWSheadline\": [\n                        \"LIGHT SNOW LIKELY LATE TONIGHT\"\n                    ],\n                    \"BLOCKCHANNEL\": [\n                        \"EAS\",\n                        \"NWEM\",\n                        \"CMAS\"\n                    ],\n                    \"EAS-ORG\": [\n                        \"WXR\"\n                    ]\n                },\n                \"scope\": \"Public\",\n                \"code\": \"IPAWSv1.0\",\n                \"language\": \"en-US\",\n                \"web\": \"http://www.weather.gov\",\n                \"eventCode\": {\n                    \"SAME\": [\n                        \"SPS\"\n                    ],\n                    \"NationalWeatherService\": [\n                        \"SPS\"\n                    ]\n                }\n            }\n        },\n        {\n            \"id\": \"https://api.weather.gov/alerts/urn:oid:2.49.0.1.840.0.b223a23810f154d96d0d97456b98216ffe2bcb9d.001.1\",\n            \"type\": \"Feature\",\n            \"geometry\": null,\n            \"properties\": {\n                \"@id\": \"https://api.weather.gov/alerts/urn:oid:2.49.0.1.840.0.b223a23810f154d96d0d97456b98216ffe2bcb9d.001.1\",\n                \"@type\": \"wx:Alert\",\n                \"id\": \"urn:oid:2.49.0.1.840.0.b223a23810f154d96d0d97456b98216ffe2bcb9d.001.1\",\n                \"areaDesc\": \"Inner waters from Point Mugu to San Mateo Pt. CA including Santa Catalina and Anacapa Islands; Outer waters from Santa Cruz Island to San Clemente Island to 60 NM offshore including San Nicolas and Santa Barbara Islands\",\n                \"geocode\": {\n                    \"SAME\": [\n                        \"057655\",\n                        \"057676\"\n                    ],\n                    \"UGC\": [\n                        \"PZZ655\",\n                        \"PZZ676\"\n                    ]\n                },\n                \"affectedZones\": [\n                    \"https://api.weather.gov/zones/forecast/PZZ655\",\n                    \"https://api.weather.gov/zones/forecast/PZZ676\"\n                ],\n                \"references\": [],\n                \"sent\": \"2025-12-03T02:03:00-08:00\",\n                \"effective\": \"2025-12-03T02:03:00-08:00\",\n                \"onset\": \"2025-12-03T21:00:00-08:00\",\n                \"expires\": \"2025-12-03T10:15:00-08:00\",\n                \"ends\": \"2025-12-04T14:00:00-08:00\",\n                \"status\": \"Actual\",\n                \"messageType\": \"Alert\",\n                \"category\": \"Met\",\n                \"severity\": \"Minor\",\n                \"certainty\": \"Likely\",\n                \"urgency\": \"Expected\",\n                \"event\": \"Small Craft Advisory\",\n                \"sender\": \"w-nws.webmaster@noaa.gov\",\n                \"senderName\": \"NWS Los Angeles/Oxnard CA\",\n                \"headline\": \"Small Craft Advisory issued December 3 at 2:03AM PST until December 4 at 2:00PM PST by NWS Los Angeles/Oxnard CA\",\n                \"description\": \"* WHAT...Hazardous sea conditions.\\n\\n* WHERE...Inner waters from Point Mugu to San Mateo Pt. CA\\nincluding Santa Catalina and Anacapa Islands and Outer waters\\nfrom Santa Cruz Island to San Clemente Island
